vi "unlock_sol.vi"() -> (3 "Boolean":bool)   [LabVIEW 2021]
panel:
  in  "error in":errorcluster
  out "error out":errorcluster
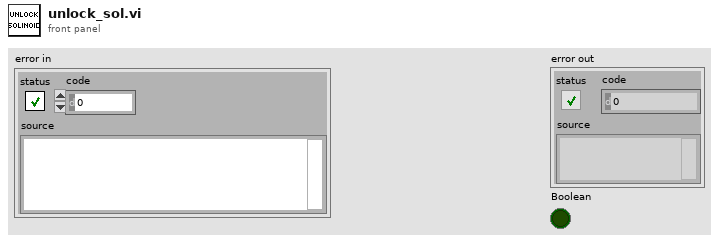
[diagram p1: front panel]
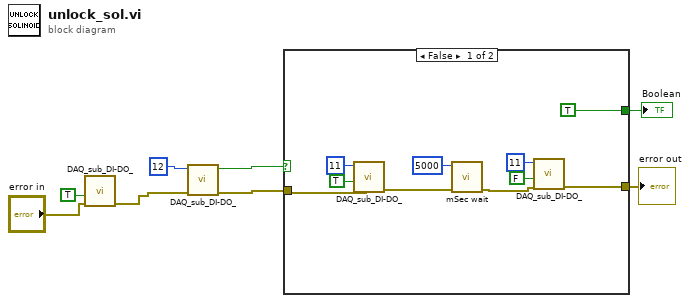
[diagram p0: block diagram]
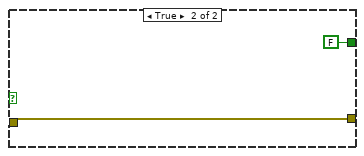
[diagram p2: hidden frame]
diagram:
  n1 = call "DAQ_sub_DI-DO_.vi"("error in"="error in", "All OFF"=TRUE) -> ("error out"=w3:errorcluster)  [unwired: 8 in, 1 out]
  n2 = call "DAQ_sub_DI-DO_.vi"("error in"=w3, "Channel"=12) -> ("error out"=w6:errorcluster, "DigitalRead"=w7:bool)  [unwired: 8 in]
  n3 = case shown="False" w7 {
    tunnel: w6 -> [w18 w20]
    tunnel: [w10 w20] -> w5
    tunnel: [TRUE FALSE] -> w4
    frame False {
      n4 = call "DAQ_sub_DI-DO_.vi"("error in"=w18, "ON/OFF"=TRUE, "Channel"=11) -> ("error out"=w13:errorcluster)  [unwired: 7 in, 1 out]
      n5 = call "mSec wait.vi"("Error in"=w13, "mSec wait"=u32 5000) -> ("Error out"=w11:errorcluster)  [unwired: 9 in]
      n6 = call "DAQ_sub_DI-DO_.vi"("error in"=w11, "ON/OFF"=FALSE, "Channel"=11) -> ("error out"=w10:errorcluster)  [unwired: 7 in, 1 out]
    }
    frame True {
    }
  }
  "error out" <- w5
  "Boolean" <- w4
